vi "Write now place.vi"(8 "error in (no error)":errorcluster, 10 "now place":cluster{"x":dbl, "y":dbl}, 11 "mainclass in":refnum<class "mainclass.lvclass">) -> (0 "error out":errorcluster, 3 "mainclass out":refnum<class "mainclass.lvclass">)   [LabVIEW 2013, in "mainclass.lvclass"]
uses:
  mainclass.lvclass
  mainclass.lvclass/mainclass.ctl
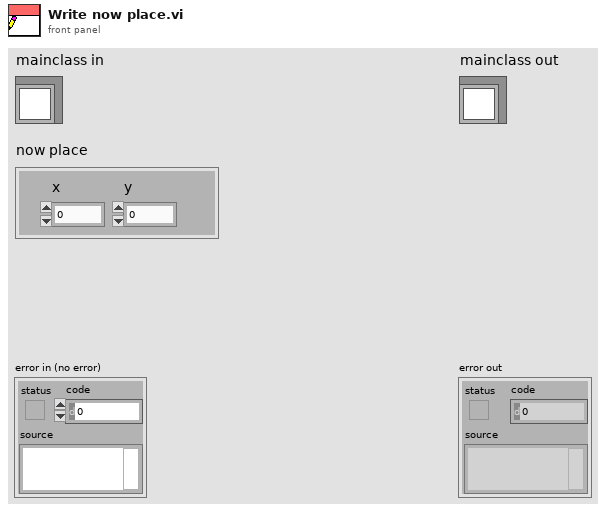
[diagram p1: front panel]
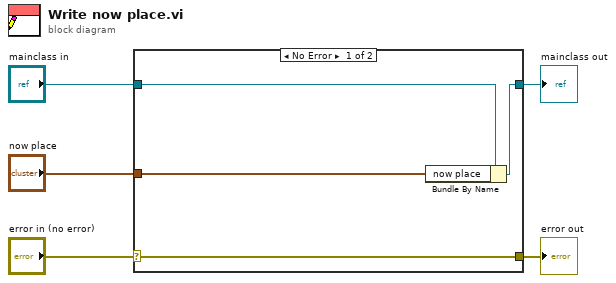
[diagram p0: block diagram]
diagram:
  n1 = case shown="No Error" "error in (no error)" {
    selector: "error in (no error)" -> [w9 w10]
    tunnel: [w9 w10] -> w4
    tunnel: [w7 w11] -> w2
    tunnel: "mainclass in" -> [w8 w11]
    tunnel: "now place" -> [w6 _]
    frame No Error {
      n2 = Bundle By Name(cluster=w8, "now place"=w6) -> (w7:refnum<class "mainclass.lvclass">)
    }
    frame Error {
    }
  }
  "error out" <- w4
  "mainclass out" <- w2
